vi "Compute Lifetime Ramp.vi"(5 "Include Infinity":bool, 7 "Include 0":bool, 8 "# Points":i32, 9 "Min Tau":ext, 10 "Max Tau":ext, 11 "Ramp Type":enum16{"Linear", "Logarithmic"}(ring)) -> (3 "Lifetime Ramp":ext[](array[numeric]))   [LabVIEW 2019]
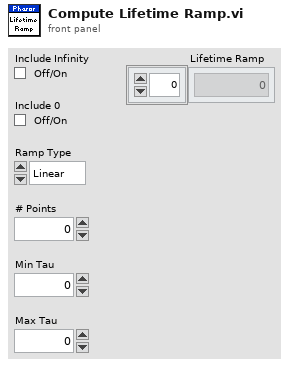
[diagram p1: front panel]
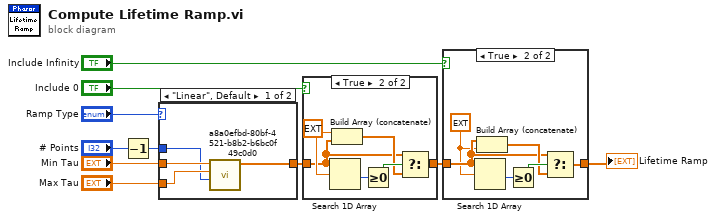
[diagram p0: block diagram]
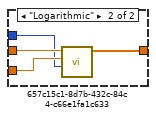
[diagram p4: hidden frame]
diagram:
  n1 = Decrement(x="# Points") -> (x-1=w1:i32)
  n2 = case shown="\"Linear\", Default" "Ramp Type" {
    tunnel: "Min Tau" -> [w14 w17]
    tunnel: "Max Tau" -> [w13 w16]
    tunnel: w1 -> [w12 w15]
    tunnel: [w11 w18] -> w5
    frame "Linear", Default {
      n3 = call "a8a0efbd-80bf-4521-b8b2-b6bc0f49c0d0.vi"("# Steps (1)"=w12, "End (1)"=w13, "Start (0)"=w14) -> ("Ramp"=w11:ext[])  [unwired: 6 in, 2 out]
    }
    frame "Logarithmic" {
      n4 = call "657c15c1-8d7b-432c-84c4-c66e1fa1c633.vi"("# Steps (1)"=w15, "End (1)"=w16, "Start (1)"=w17) -> ("Ramp"=w18:ext[])  [unwired: 7 in, 1 out]
    }
  }
  n5 = case shown="True" "Include 0" {
    tunnel: w5 -> [w19 w21]
    tunnel: [w19 w20] -> w7
    frame False {
    }
    frame True {
      w23 = ext 0.0 ("element")
      n6 = Search 1D Array(1D array=w21, element=w23) -> (index of element=w25:i32)  [unwired: 1 in]
      n7 = Build Array (concatenate)(w23, w21) -> (w22:ext[])
      n8 = Greater Or Equal To 0?(x=w25) -> (x >= 0?=w24:bool)
      n9 = Select(t=w21, s=w24, f=w22) -> (s? t:f=w20:ext[])
    }
  }
  n10 = case shown="True" "Include Infinity" {
    tunnel: w7 -> [w26 w29]
    tunnel: [w26 w28] -> w9
    frame False {
    }
    frame True {
      w27 = ext inf ("element")
      n11 = Search 1D Array(1D array=w29, element=w27) -> (index of element=w32:i32)  [unwired: 1 in]
      n12 = Build Array (concatenate)(w29, w27) -> (w30:ext[])
      n13 = Greater Or Equal To 0?(x=w32) -> (x >= 0?=w31:bool)
      n14 = Select(t=w29, s=w31, f=w30) -> (s? t:f=w28:ext[])
    }
  }
  "Lifetime Ramp" <- w9
